vi "Get Ref.vi"(8 "error in":errorcluster, 11 "Hanlde Out":T2) -> (0 "error out":errorcluster, 2 "FPGA Ref":T1, 3 "Handle Out":T2)   [LabVIEW 2017, in "FPGA Session.lvclass"]
uses:
  FPGA Session.lvclass
  <vilib>/MSR Consulting, LLC/General Reuse/Session APIs/_Session Fwk/Typedefs/Session Handle.ctl
  <vilib>/MSR Consulting, LLC/General Reuse/Session APIs/_Session Fwk/Session - Root.lvclass
  FPGA Ref.ctl
  FPGA Session.lvclass/FPGA Session.ctl
  Read FPGA Ref.vi
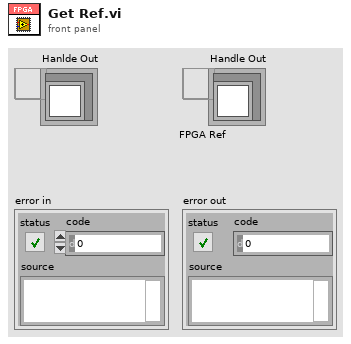
[diagram p1: front panel]
types:
  T1 = typedef "FPGA Ref.ctl" = refnum<k20>
  T2 = typedef "Session - Root.lvclass/Session Handle.ctl" = refnum<data-value>
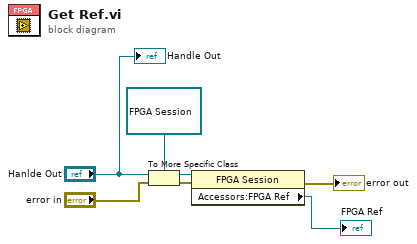
[diagram p0: block diagram]
diagram:
  n1 = To More Specific Class(target class=refnum<data-value> refnum ("Hanlde Out"), reference="Hanlde Out", error in="error in") -> (specific class reference=w6:refnum<data-value>, error out=w4:errorcluster)
  n2 = property class="FPGA Session"(reference=w6, error in=w4) -> (error out=→"error out":errorcluster, "Accessors:FPGA Ref"=→"FPGA Ref":T1)  [unwired: 1 out]
  "Handle Out" <- "Hanlde Out"
